vi "AE Acquisition.vi"(7 "Action":T1, 8 "error in (no error)":errorcluster, 10 "Freq":i32, 11 "DataPath":path) -> (0 "error out":errorcluster, 1 "Period(ms)":i32, 2 "Freq Out":i32, 3 "DataPath Out":path)   [LabVIEW 2013, in "main.lvlib"]
uses:
  main.lvlib
  Controls/Enum Globals.ctl
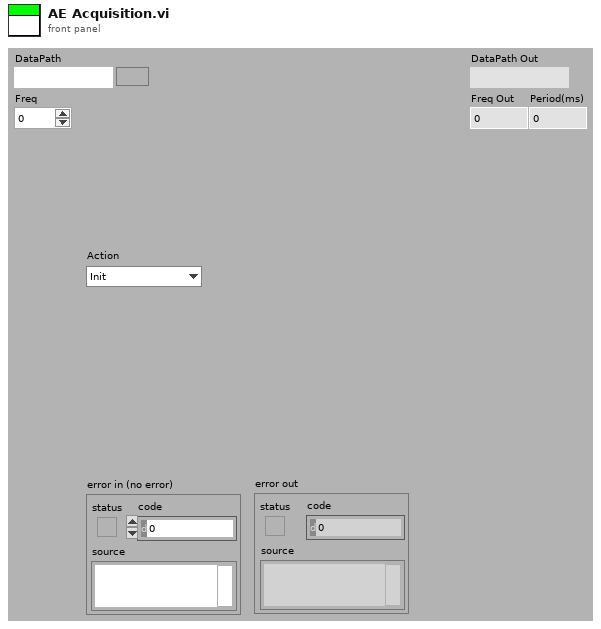
[diagram p1: front panel]
types:
  T1 = typedef "main.lvlib/Enum Globals.ctl" = enum16{"Init", "Set DataPath", "Set Freq", "Get"}
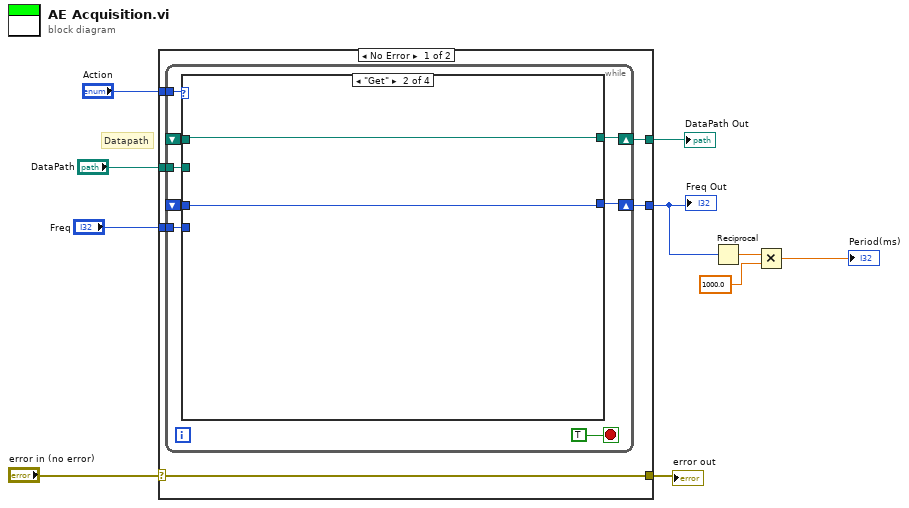
[diagram p0: block diagram]
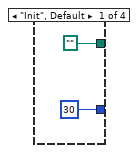
[diagram p2: hidden frame]
diagram:
  # "Datapath"
  n1 = case shown="No Error" "error in (no error)" {
    selector: "error in (no error)" -> [w16 w35]
    tunnel: [w16 w35] -> w9
    tunnel: "Action" -> [w15 _]
    tunnel: "DataPath" -> [w14 w34]
    tunnel: "Freq" -> [w13 w33]
    tunnel: [w12 w34] -> w5
    tunnel: [w11 w33] -> w4
    frame No Error {
      n2 = while {
        tunnel: w15 -> [w23]
        shift-right: [w22] -> w12
        shift-left: _ -> [w21]
        tunnel: w14 -> [w20]
        shift-right: [w19] -> w11
        shift-left: _ -> [w18]
        tunnel: w13 -> [w17]
        stop <- TRUE stop-if-true
        n3 = case shown="\"Get\"" w23 {
          tunnel: [path "" w27 w30 w32] -> w22
          tunnel: w21 -> [_ w27 _ w32]
          tunnel: w20 -> [_ _ w30 _]
          tunnel: [30 w28 w29 w31] -> w19
          tunnel: w18 -> [_ w28 w29 _]
          tunnel: w17 -> [_ _ _ w31]
          frame "Init", Default {
          }
          frame "Get" {
          }
          frame "Set DataPath" {
          }
          frame "Set Freq" {
          }
        }
      }
    }
    frame Error {
    }
  }
  "error out" <- w9
  "DataPath Out" <- w5
  "Freq Out" <- w4
  n4 = Reciprocal(x=w4) -> (1/x=w3:dbl)
  n5 = Multiply(x=w3, y=1000.0) -> (x*y=→"Period(ms)":dbl)
